vi "parse_uint16.vi"   [LabVIEW 2014]
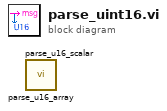
[diagram p0: block diagram]
diagram:
  n1 = call "parse_u16_array.vi"() -> ()  [unwired: 5 in, 3 out]
  n2 = call "parse_u16_scalar.vi"() -> ()  [unwired: 5 in, 3 out]
